vi "get_price.vi"(8 "error in (no error)":errorcluster, 11 "Chair in":refnum<class "Chair.lvclass">) -> (0 "error out":errorcluster, 2 "price":dbl, 3 "Chair out":refnum<class "Chair.lvclass">)   [LabVIEW 2021, in "Chair.lvclass"]
uses:
  Chair.lvclass
  Chair.lvclass/Chair.ctl
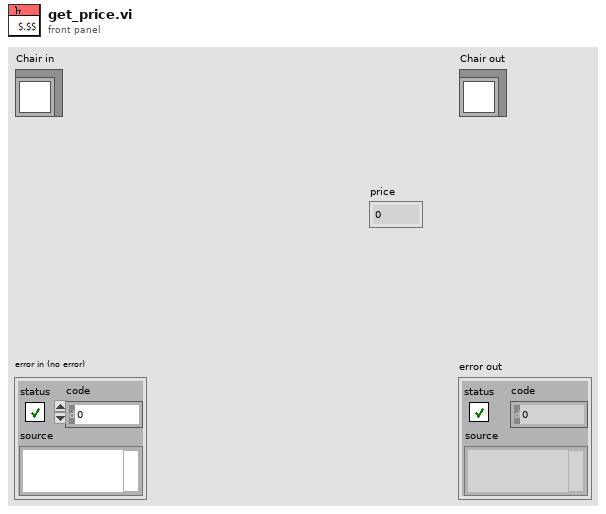
[diagram p1: front panel]
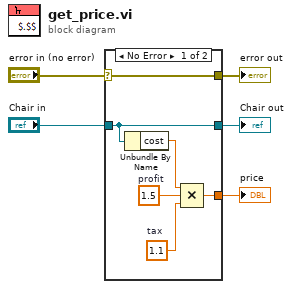
[diagram p0: block diagram]
diagram:
  n1 = case shown="No Error" "error in (no error)" {
    selector: "error in (no error)" -> [w11 w13]
    tunnel: [w11 w13] -> w1
    tunnel: [w10 w12] -> w4
    tunnel: "Chair in" -> [w10 w12]
    tunnel: [w6 _] -> w3
    frame No Error {
      w7 = 1.1  # tax
      w8 = 1.5  # profit
      n2 = Unbundle By Name(w10) -> ("cost"=w9:dbl)
      n3 = Compound Arithmetic op=MULTIPLY(w9, w8, w7) -> (w6:dbl)
    }
    frame Error {
    }
  }
  "error out" <- w1
  "Chair out" <- w4
  "price" <- w3
